vi "Measurement UI.vi"() -> ()   [LabVIEW 2020, in "NI-DMM Measurement.lvlib"]
uses:
  NI-DMM Measurement.lvlib
panel:
  in  "measurement_type":i32(ring)=1 caption="Measurement type" items=["DC Volts"=1, "AC Volts"=2, "DC Current"=3, "AC Current"=4, "2-Wire Resistance"=5, "4-Wire Resistance"=101, "Frequency"=104, "Period"=105, "AC Volts DC Coupled"=1001, "Diode"=1002, "Waveform Voltage"=1003, "Waveform Current"=1004, "Capacitance"=1005, "Inductance"=1006, "Temperature"=108]
  in  "pin_name":string="Pin1" caption="Pin name"
  out "absolute_resolution":dbl caption="Absolute resolution" format="%_3p"
  out "signal_out_of_range":bool caption="Signal out of range"
  out "measured_value":dbl caption="Measured value" format="%.6f"
  in  "resolution_digits":dbl=5.5 caption="Resolution (digits)" format="%.1f"
  in  "range":dbl=10.0 caption="Range" format="%.2p"
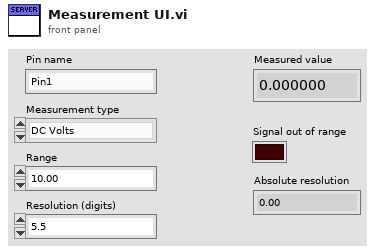
[diagram p1: front panel]
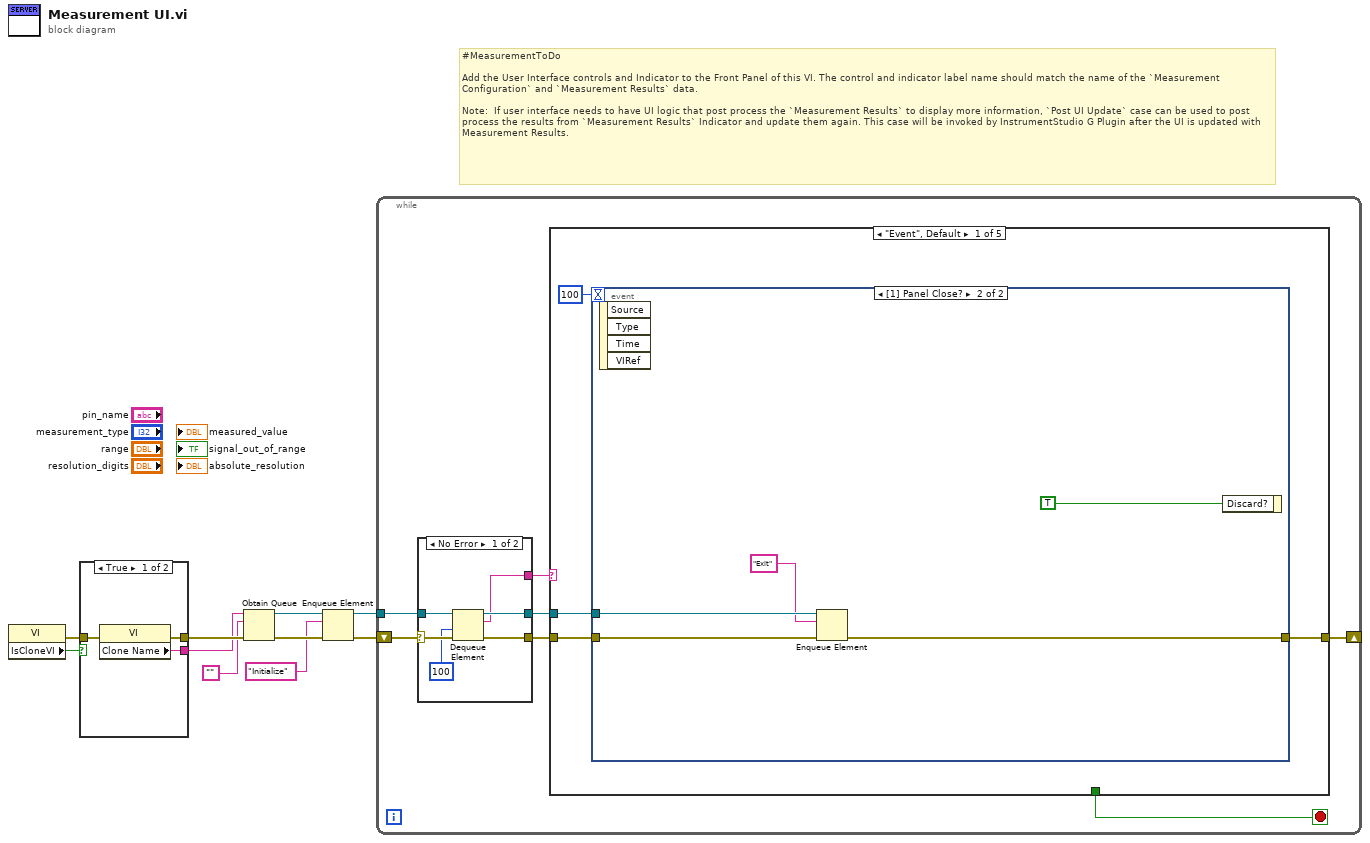
[diagram p0: block diagram]
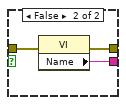
[diagram p2: hidden frame]
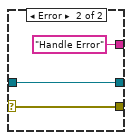
[diagram p3: hidden frame]
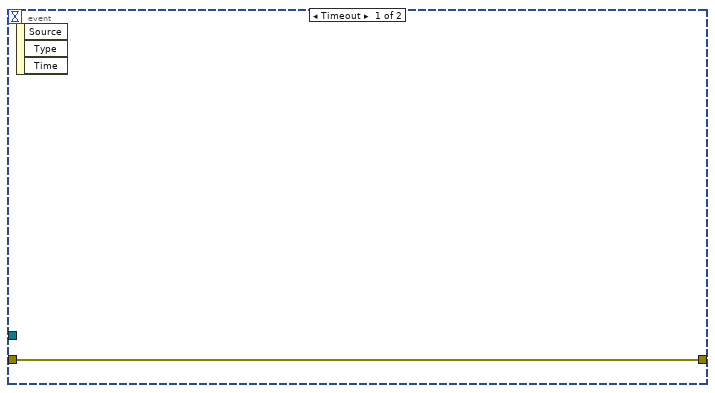
[diagram p4: hidden frame]
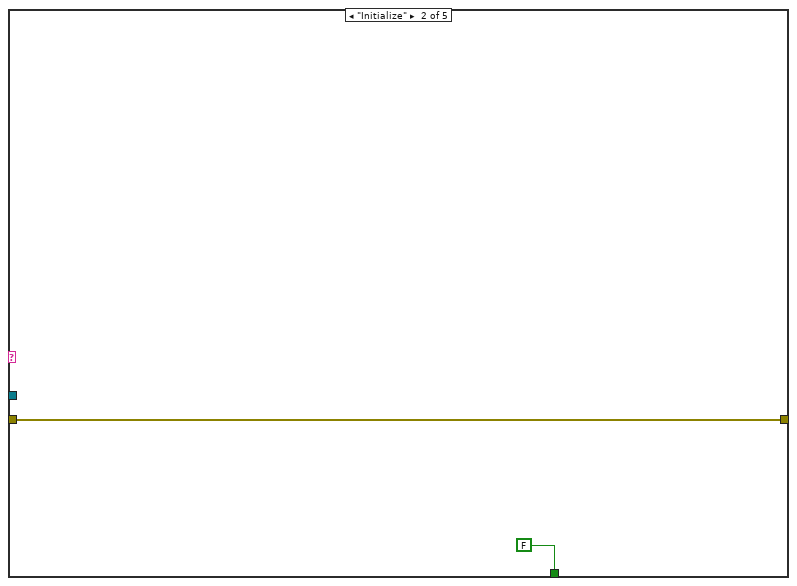
[diagram p5: hidden frame]
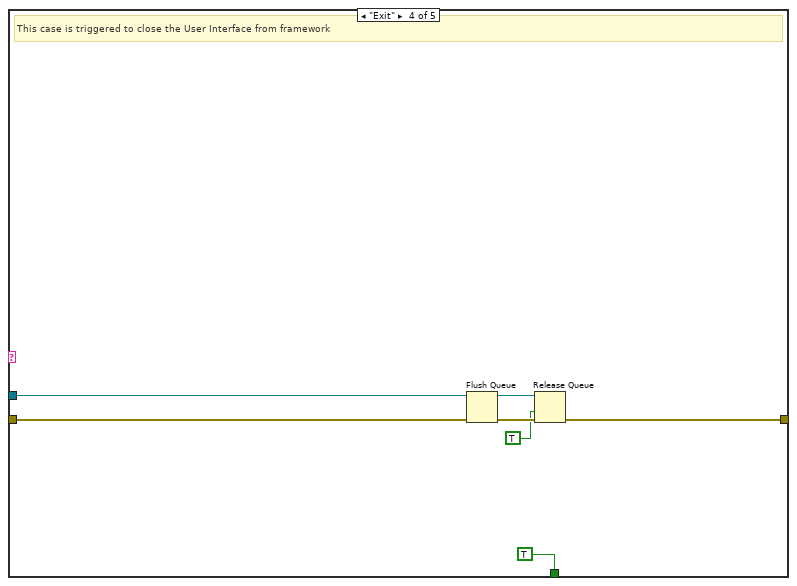
[diagram p7: hidden frame]
diagram:
  # "#MeasurementToDo  \n\nAdd the User Interface controls and Indicator to the Front Panel of this VI. The control and indicator label name should match the name of the `Measurement Configuration` and `Measurement Results` data.\n\nNote:  If user interface needs to have UI logic that post process the `Measurement Results` to display more information, `Post UI Update` case can be used to post process the results from `Measurement Results` Indicator and update them again. This case will be invoked by InstrumentStudio G Plugin after the UI is updated with Measurement Results."
  n1 = property class="VI"() -> (error out=w1:errorcluster, "IsCloneVI"=w2:bool)  [unwired: 2 in, 1 out]
  n2 = case shown="True" w2 {
    tunnel: [w13 w16] -> w10
    tunnel: [w12 w15] -> w9
    tunnel: w1 -> [w11 w14]
    frame True {
      n3 = property class="VI"(error in=w11) -> (error out=w13:errorcluster, "Clone Name"=w12:string)  [unwired: 1 in, 1 out]
    }
    frame False {
      n4 = property class="VI"(error in=w14) -> (error out=w16:errorcluster, "Name"=w15:string)  [unwired: 1 in, 1 out]
    }
  }
  n5 = Obtain Queue(name (unnamed)=w9, element data type="", error in (no error)=w10) -> (queue out=w6:refnum<queue>, error out=w8:errorcluster)  [unwired: 2 in, 1 out]
  n6 = Enqueue Element(queue=w6, element="Initialize", error in (no error)=w8) -> (queue out=w5:refnum<queue>, error out=w7:errorcluster)  [unwired: 1 in, 1 out]
  n7 = while {
    shift-right: [w18] -> _
    shift-left: w7 -> [w23]
    tunnel: w5 -> [w21]
    stop <- w17 stop-if-true
    n8 = case shown="No Error" w23 {
      selector: w23 -> [w29 w32]
      tunnel: [w28 w32] -> w22
      tunnel: w21 -> [w27 w31]
      tunnel: [w26 w31] -> w20
      tunnel: [w25 "Handle Error"] -> w19
      frame No Error {
        n9 = Dequeue Element(queue=w27, timeout in ms (-1)=100, error in (no error)=w29) -> (queue out=w26:refnum<queue>, element=w25:string, error out=w28:errorcluster)  [unwired: 1 out]
      }
      frame Error {
      }
    }
    n10 = case shown="\"Event\", Default" w19 {
      tunnel: w22 -> [w35 w44 w45 w52 w53]
      tunnel: w20 -> [w33 _ _ w50 _]
      tunnel: [w36 w44 w45 w47 w53] -> w18
      tunnel: [_ FALSE _ TRUE _] -> w17
      frame "Event", Default {
        n11 = event shown="[1] Panel Close?" {
          selector: _ -> [_ _]
          dyn-events: _ -> [_ _]
          timeout: 100 -> [_ _]
          tunnel: [w37 w40] -> w36
          tunnel: w35 -> [w37 w41]
          tunnel: w33 -> [_ w39]
          event Timeout {
            n12 = event-data() -> ()  [unwired: 1 in, 3 out]
          }
          event Panel Close? {
            n13 = event-data() -> ()  [unwired: 1 in, 4 out]
            n14 = Enqueue Element(queue=w39, element="Exit", error in (no error)=w41) -> (error out=w40:errorcluster)  [unwired: 1 in, 2 out]
            n15 = event-data("Discard?"=TRUE) -> ()  [unwired: 1 in, 1 out]
          }
        }
      }
      frame "Initialize" {
      }
      frame "Post UI Update" {
        # "This case will be triggered, after framework updates the User interface with result values."
      }
      frame "Exit" {
        # "This case is triggered to close the User Interface from framework"
        n16 = Flush Queue(queue=w50, error in (no error)=w52) -> (queue out=w49:refnum<queue>, error out=w48:errorcluster)  [unwired: 1 out]
        n17 = Release Queue(queue=w49, force destroy? (F)=TRUE, error in (no error)=w48) -> (error out=w47:errorcluster)  [unwired: 2 out]
      }
      frame "Handle Error" {
      }
    }
  }
